vi "Tri_sub.vi"(0 "E1":dbl[](array[numeric]), 1 "E2":dbl[](array[numeric]), 2 "O0":dbl[](array[numeric]), 3 "O1":dbl[](array[numeric]), 4 "V0":dbl[](array[numeric])) -> (5 "Collision?":bool)   [LabVIEW 2011]
uses:
  <vilib>/Analysis/baseanly.llb/Real Dot Product.vi
  <vilib>/Analysis/NI_AALBase.lvlib
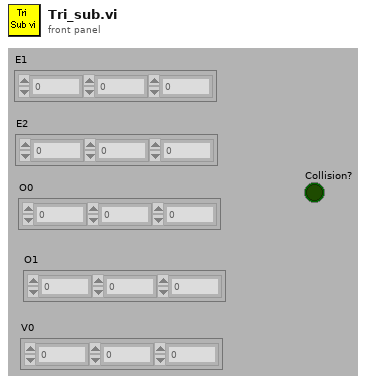
[diagram p1: front panel]
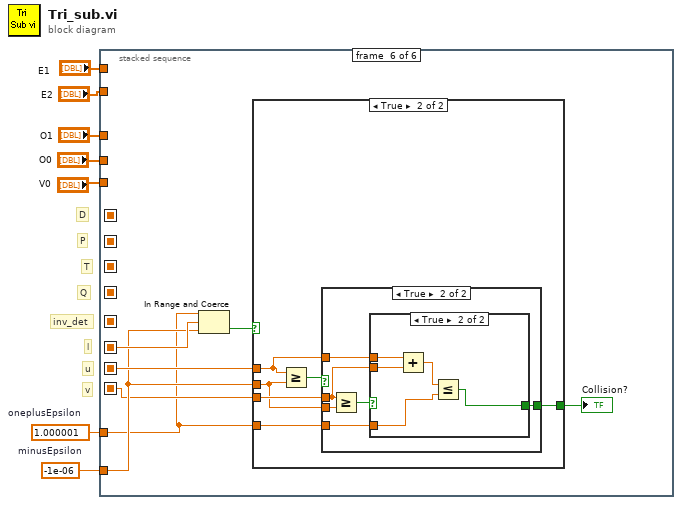
[diagram p0: block diagram]
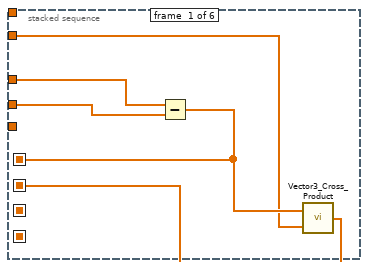
[diagram p2: hidden frame]
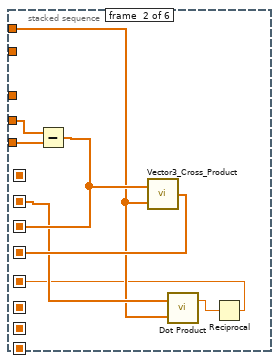
[diagram p3: hidden frame]
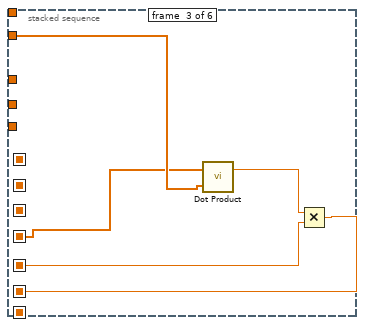
[diagram p4: hidden frame]
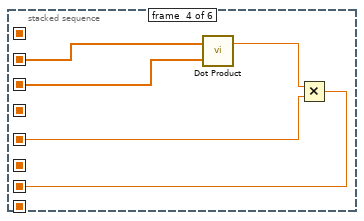
[diagram p5: hidden frame]
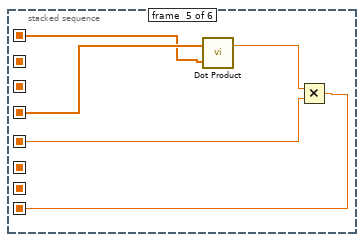
[diagram p6: hidden frame]
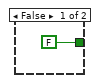
[diagram p7: hidden frame]
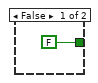
[diagram p8: hidden frame]
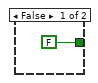
[diagram p9: hidden frame]
diagram:
  w1 = 1.000001  # oneplusEpsilon
  w2 = -1e-06  # minusEpsilon
  # "v"
  # "u"
  # "l"
  # "inv_det"
  # "Q"
  # "T"
  # "P"
  # "D"
  n1 = stacked-sequence {
    seq-local: [w10 _ _ _ _ _] -> [_ _ _ _ w31 _]
    seq-local: [w8 _ _ _ _ _] -> [_ w16 _ w28 _ _]
    seq-local: [_ w18 _ _ _ _] -> [_ _ _ w27 _ _]
    seq-local: [_ w17 _ _ _ _] -> [_ _ w24 _ w32 _]
    seq-local: [_ w13 _ _ _ _] -> [_ _ w23 w30 w35 _]
    seq-local: [_ _ w21 _ _ _] -> [_ _ _ _ _ w42]
    seq-local: [_ _ _ w26 _ _] -> [_ _ _ _ _ w40]
    seq-local: [_ _ _ _ w33 _] -> [_ _ _ _ _ w38]
    tunnel: "O1" -> [w12 _ _ _ _ _]
    tunnel: "O0" -> [w11 w20 _ _ _ _]
    tunnel: "E2" -> [w9 _ w25 _ _ _]
    tunnel: "V0" -> [_ w19 _ _ _ _]
    tunnel: "E1" -> [_ w15 _ _ _ _]
    tunnel: w2 -> [_ _ _ _ _ w39]
    tunnel: w1 -> [_ _ _ _ _ w36]
    frame #0 {
      n2 = Subtract(x=w12, y=w11) -> (x-y=w10:dbl[])
      n3 = call "Vector3_Cross_Product.vi"("V"=w9, "U"=w10) -> ("UxV"=w8:dbl[])
    }
    frame #1 {
      n4 = Subtract(x=w20, y=w19) -> (x-y=w18:dbl[])
      n5 = call "Vector3_Cross_Product.vi"("V"=w15, "U"=w18) -> ("UxV"=w17:dbl[])
      n6 = call-poly <vilib>:"Dot Product.vi"("Y Vector"=w15, "X Vector"=w16) -> ("X * Y"=w14:dbl)  [unwired: 1 out]
      n7 = Reciprocal(x=w14) -> (1/x=w13:dbl)
    }
    frame #2 {
      n8 = call-poly <vilib>:"Dot Product.vi"("Y Vector"=w25, "X Vector"=w24) -> ("X * Y"=w22:dbl)  [unwired: 1 out]
      n9 = Multiply(x=w22, y=w23) -> (x*y=w21:dbl)
    }
    frame #3 {
      n10 = call-poly <vilib>:"Dot Product.vi"("Y Vector"=w27, "X Vector"=w28) -> ("X * Y"=w29:dbl)  [unwired: 1 out]
      n11 = Multiply(x=w29, y=w30) -> (x*y=w26:dbl)
    }
    frame #4 {
      n12 = call-poly <vilib>:"Dot Product.vi"("Y Vector"=w31, "X Vector"=w32) -> ("X * Y"=w34:dbl)  [unwired: 1 out]
      n13 = Multiply(x=w34, y=w35) -> (x*y=w33:dbl)
    }
    frame #5 {
      n14 = In Range and Coerce(upper limit=w36, x=w42, lower limit=w39) -> (In Range?=w41:bool)  [unwired: 1 out]
      n15 = case shown="True" w41 {
        tunnel: w40 -> [_ w46]
        tunnel: w39 -> [_ w47]
        tunnel: w38 -> [_ w48]
        tunnel: w36 -> [_ w45]
        tunnel: [FALSE w44] -> w37
        frame False {
        }
        frame True {
          n16 = Greater Or Equal?(x=w46, y=w47) -> (x >= y?=w49:bool)
          n17 = case shown="True" w49 {
            tunnel: w48 -> [_ w53]
            tunnel: w47 -> [_ w56]
            tunnel: w46 -> [_ w54]
            tunnel: w45 -> [_ w52]
            tunnel: [FALSE w51] -> w44
            frame False {
            }
            frame True {
              n18 = Greater Or Equal?(x=w53, y=w56) -> (x >= y?=w55:bool)
              n19 = case shown="True" w55 {
                tunnel: w54 -> [_ w62]
                tunnel: w53 -> [_ w61]
                tunnel: w52 -> [_ w59]
                tunnel: [FALSE w58] -> w51
                frame False {
                }
                frame True {
                  n20 = Add(x=w62, y=w61) -> (x+y=w60:dbl)
                  n21 = Less Or Equal?(x=w60, y=w59) -> (x <= y?=w58:bool)
                }
              }
            }
          }
        }
      }
      "Collision?" <- w37
    }
  }
